vi "五参数水样测试.vi"(11 "启动参数":T1={"测量模式"=enum."水样测试", "数据标记表"="N", "测量时间"=3.0}) -> ()   [LabVIEW 2016, in "斯坦道仪器.lvlib"]
uses:
  PLC/PLC.lvlib
panel:
  out "枚举":T2(ring)
  out "状态":string
  out "数值":i32
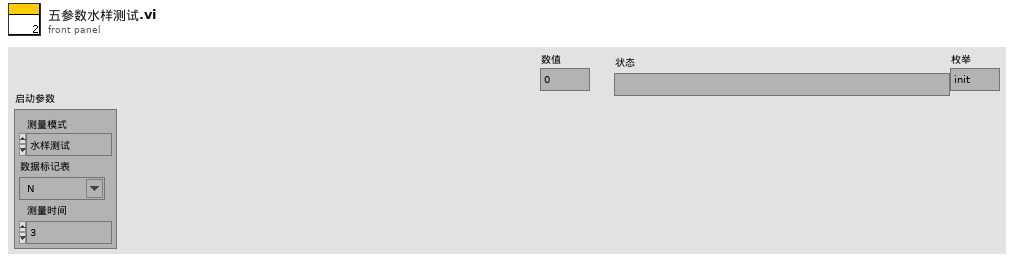
[diagram p1: front panel]
types:
  T1 = cluster{"测量模式":enum16{"待机", "水样测试", "标样核查", "零点核查", "跨度核查", "空白测试", "平行样测试", "加标回收", "空白校准", "标样校准", "初始化（清洗）"}, "数据标记表":string, "测量时间":dbl}
  T2 = enum16{"init", "开机", "启动测量", "读取测量值", "存储数据", "关闭测量", "关机", "结束"}
  T3 = cluster{"时间标识":timestamp, "设备":string, "日志信息":string, "流程参数":string}
  T4 = cluster{"starting address":u16, "holding register value":u16}
  T5 = enum16{"idle", "init", "读状态", "读参数", "多个写入", "单个写入", "线圈写入"}
  T6 = enum16{"待机", "水样测试", "标样核查", "零点核查", "跨度核查", "空白测试", "平行样测试", "加标回收", "空白校准", "标样校准", "初始化（清洗）"}
  T7 = cluster{"水温":dbl, "pH":dbl, "DO":dbl, "Cond":dbl, "Turb":dbl, "叶绿素":dbl, "藻密度":dbl, "蓝绿藻":dbl, "ORP":dbl, "NH3N":dbl}
  T8 = cluster{"数据标记表":string, "测量模式":enum16{"待机", "水样测试", "标样核查", "零点核查", "跨度核查", "空白测试", "平行样测试", "加标回收", "空白校准", "标样校准", "初始化（清洗）"}, "database":string}
  T9 = cluster{"因子编码":string, "单位":string, "标样参考值":sgl, "水样数据时间":timestamp, "水样实测值":sgl, "水样数据标识":string, "K":sgl, "B":sgl, "T":sgl, "H":sgl, "水深":sgl}
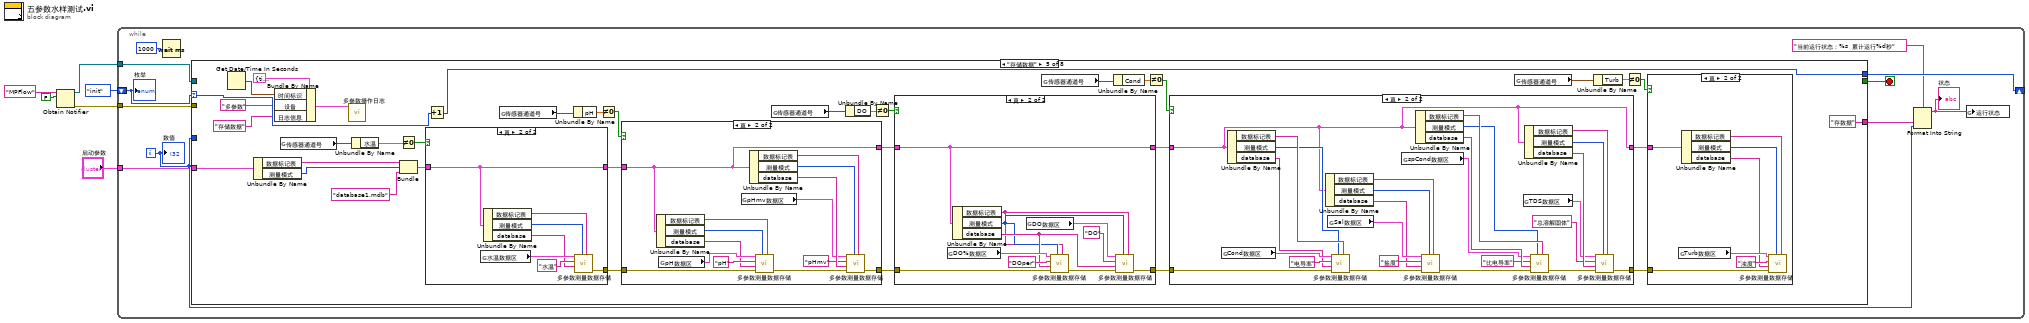
[diagram p0: block diagram]
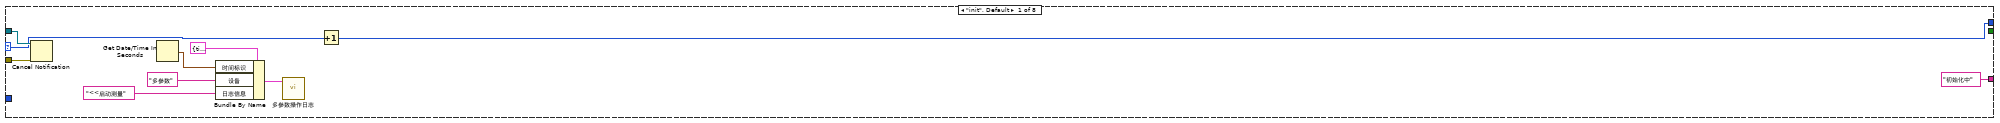
[diagram p2: hidden frame]
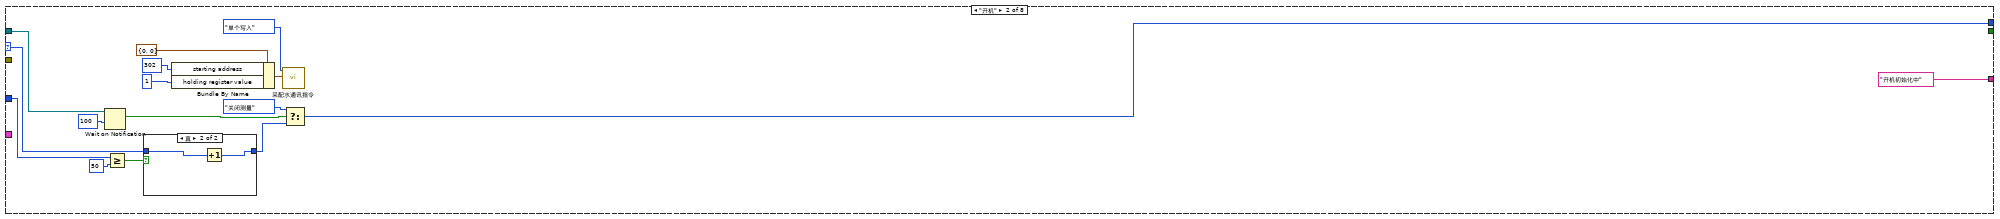
[diagram p3: hidden frame]
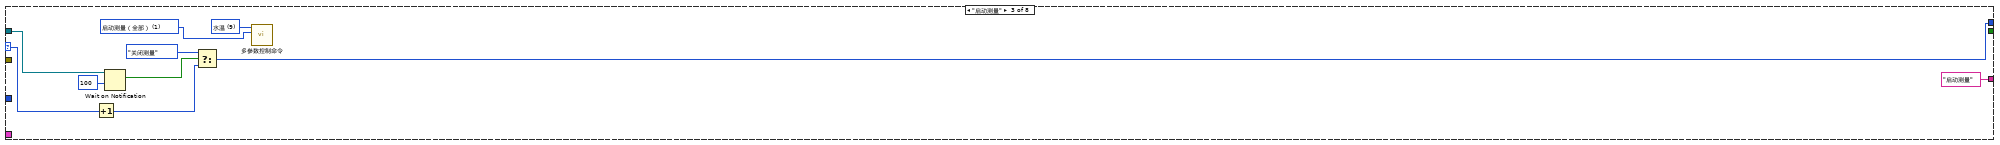
[diagram p5: hidden frame]
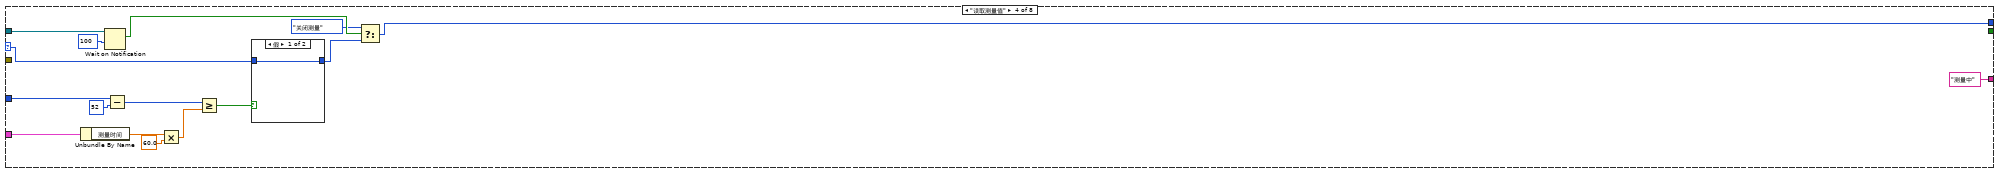
[diagram p6: hidden frame]
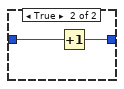
[diagram p7: hidden frame]
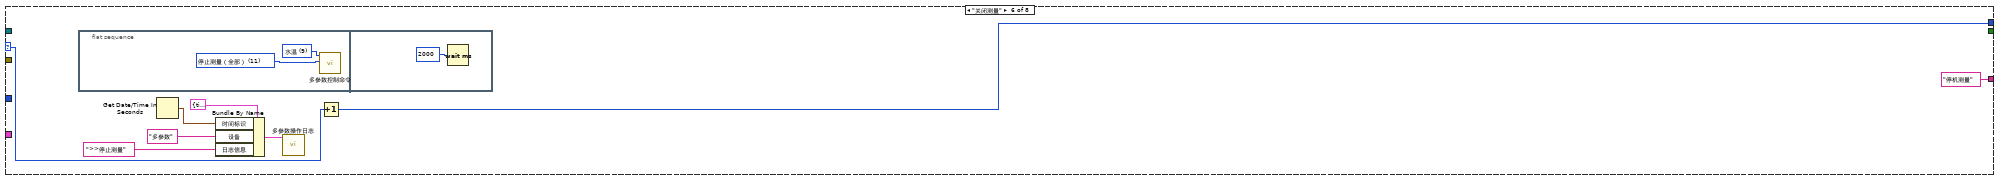
[diagram p13: hidden frame]
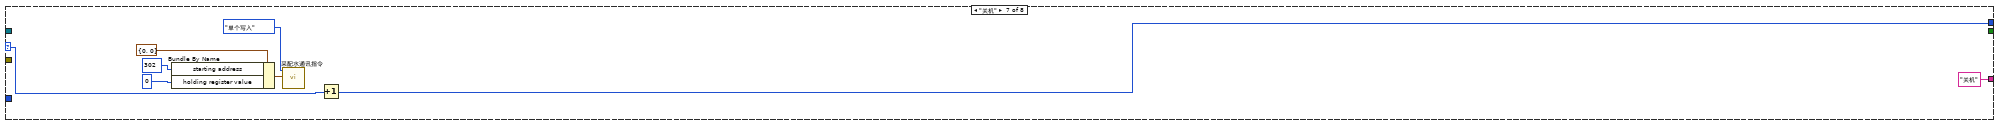
[diagram p14: hidden frame]
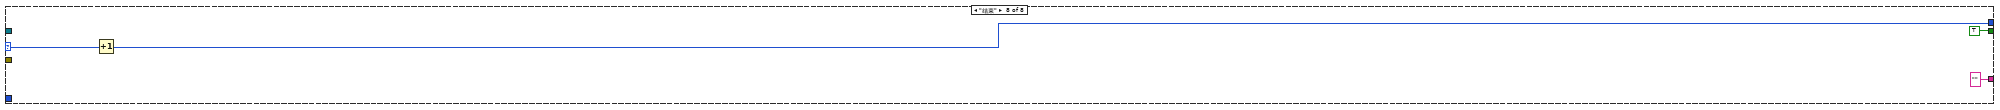
[diagram p15: hidden frame]
diagram:
  n1 = Obtain Notifier(name (unnamed)="MPFlow" ("名称（未命名）"), notification data type=FALSE) -> (notifier out=w3:refnum<notifier>, error out=w2:errorcluster)  [unwired: 2 in, 1 out]
  n2 = while {
    shift-right: [w13] -> _
    shift-left: T2."init" ("枚举") -> [w17]
    tunnel: w3 -> [w15]
    tunnel: w2 -> [w14]
    tunnel: "启动参数" -> [w7]
    i -> [w9]
    stop <- w16 stop-if-true
    n3 = Wait (ms)(milliseconds to wait=u32 1000 ("等待时间（毫秒）")) -> ()  [unwired: 1 out]
    n4 = case shown="\"存储数据\"" w17 {
      selector: w17 -> [w25 w38 w56 w72 w111 w188 w194 w202]
      tunnel: [_ _ _ _ _ _ _ TRUE] -> w16
      tunnel: w15 -> [w27 w33 w55 w69 _ _ _ _]
      tunnel: w14 -> [w26 _ _ _ _ _ _ _]
      tunnel: [w24 w31 w52 w67 w110 w187 w193 w201] -> w13
      tunnel: w9 -> [_ w37 _ w59 _ _ _ _]
      tunnel: ["初始化中" ("状态") "开机初始化中" ("状态") "启动测量" ("状态") "测量中" ("状态") "存数据" ("状态") "停机测量" ("状态") "关机" ("状态") "" ("状态")] -> w10
      tunnel: w7 -> [_ _ _ w63 w108 _ _ _]
      frame "init", Default {
        n5 = Cancel Notification(0:w27, 3:w26) -> ()  [unwired: 3 out]
        n6 = Get Date/Time In Seconds() -> (seconds since 1Jan1904=w21:timestamp)
        n7 = Bundle By Name(cluster=T3 {"时间标识"=timestamp(0 s since 1904-01-01), "设备"="", "日志信息"="", "流程参数"=""} ("data in"), "时间标识"=w21, "设备"="多参数", "日志信息"="<<启动测量") -> (w20:T3)
        n8 = call "多参数操作日志.vi"("data in"=w20) -> ()  [unwired: 10 in, 1 out]
        n9 = Increment(x=w25) -> (x+1=w24:T2)
      }
      frame "开机" {
        n10 = Wait on Notification(notifier=w33, timeout in ms (-1)=100 ("超时毫秒(-1)")) -> (notification=w34:bool)  [unwired: 2 in, 3 out]
        n11 = Greater Or Equal?(x=w37, y=50) -> (x >= y?=w35:bool)
        n12 = case shown="真" w35 {
          tunnel: w38 -> [w44 w46]
          tunnel: [w44 w45] -> w32
          frame False {
          }
          frame True {
            n13 = Increment(x=w46) -> (x+1=w45:T2)
          }
        }
        n14 = Bundle By Name(cluster=T4 {"starting address"=0, "holding register value"=0}, "starting address"=u16 302, "holding register value"=u16 1) -> (w41:T4)
        n15 = call "采配水通讯指令.vi"("数据"=w41, "命令"=T5."单个写入") -> ()  [unwired: 10 in]
        n16 = Select(t=T2."关闭测量" ("枚举"), s=w34, f=w32) -> (s? t:f=w31:T2)
      }
      frame "启动测量" {
        w47 = u16 1 items=["启动测量（全部）"=1, "初始化（清洗）"=10, "停止测量（全部）"=11, "校时"=13, "启动测量（单个传感器）"=19, "停止测量（单个传感器）"=20] ("控制命令")
        w48 = u16 9 items=["氨氮"=3, "水温"=9, "pH值"=10, "溶解氧"=11, "电导率"=12, "浊度"=13, "叶绿素a"=14, "藻密度"=15, "蓝绿藻"=16, "氧化还原电位"=17, "溶解氧%"=18, "盐度"=19] ("站号")
        n17 = Increment(x=w56) -> (x+1=w53:T2)
        n18 = Wait on Notification(notifier=w55, timeout in ms (-1)=100 ("超时毫秒(-1)")) -> (notification=w54:bool)  [unwired: 2 in, 3 out]
        n19 = Select(t=T2."关闭测量" ("枚举"), s=w54, f=w53) -> (s? t:f=w52:T2)
        n20 = call "多参数控制命令.vi"("控制命令"=w47, "站号"=w48) -> ()  [unwired: 9 in, 1 out]
      }
      frame "读取测量值" {
        n21 = Unbundle By Name(w63) -> ("测量时间"=w62:dbl)
        n22 = Wait on Notification(notifier=w69, timeout in ms (-1)=100 ("超时毫秒(-1)")) -> (notification=w70:bool)  [unwired: 2 in, 3 out]
        n23 = Subtract(x=w59, y=52) -> (x-y=w58:i32)
        n24 = Multiply(x=w62, y=60.0) -> (x*y=w60:dbl)
        n25 = Greater Or Equal?(x=w58, y=w60) -> (x >= y?=w71:bool)
        n26 = case shown="假" w71 {
          tunnel: w72 -> [w73 w75]
          tunnel: [w73 w74] -> w68
          frame False {
          }
          frame True {
            n27 = Increment(x=w75) -> (x+1=w74:T2)
          }
        }
        n28 = Select(t=T2."关闭测量" ("枚举"), s=w70, f=w68) -> (s? t:f=w67:T2)
      }
      frame "存储数据" {
        n29 = Get Date/Time In Seconds() -> (seconds since 1Jan1904=w79:timestamp)
        n30 = Unbundle By Name(w108) -> ("数据标记表"=w87:string, "测量模式"=w86:T6)
        n31 = Bundle By Name(cluster=T3 {"时间标识"=timestamp(0 s since 1904-01-01), "设备"="", "日志信息"="", "流程参数"=""} ("data in"), "时间标识"=w79, "设备"="多参数", "日志信息"="存储数据") -> (w78:T3)
        n32 = global read "多参数全局变量.vi" "传感器通道号"() -> (w103:T7)
        n33 = call "多参数操作日志.vi"("data in"=w78) -> ()  [unwired: 10 in, 1 out]
        n34 = Unbundle By Name(w103) -> ("水温"=w102:dbl)
        n35 = Not Equal To 0?(x=w102) -> (x != 0?=w101:bool)
        n36 = Bundle("数据标记表"=w87, "测量模式"=w86, "database"="database1.mdb") -> (w85:T8)  [unwired: 1 in]
        n37 = case shown="真" w101 {
          tunnel: [_ w178] -> w107
          tunnel: w85 -> [w173 w177]
          tunnel: [w173 w177] -> w84
          frame False {
          }
          frame True {
            n38 = global read "多参数全局变量.vi" "水温数据区"() -> (w180:T9)
            n39 = Unbundle By Name(w177) -> ("数据标记表"=w176:string, "测量模式"=w175:T6, "database"=w174:string)
            n40 = call "多参数测量数据存储.vi"("数据标记表"=w176, "测量模式"=w175, "database"=w174, "table输入"="水温", "data in"=w180) -> ("error out"=w178:errorcluster)  [unwired: 6 in]
          }
        }
        n41 = Increment(x=w111) -> (x+1=w110:T2)
        n42 = global read "多参数全局变量.vi" "传感器通道号"() -> (w96:T7)
        n43 = Unbundle By Name(w96) -> ("pH"=w95:dbl)
        n44 = Not Equal To 0?(x=w95) -> (x != 0?=w100:bool)
        n45 = case shown="真" w100 {
          tunnel: w107 -> [_ w172]
          tunnel: [_ w161] -> w106
          tunnel: w84 -> [w158 w166]
          tunnel: [w158 w166] -> w82
          frame False {
          }
          frame True {
            n46 = Unbundle By Name(w166) -> ("数据标记表"=w169:string, "测量模式"=w168:T6, "database"=w167:string)
            n47 = global read "多参数全局变量.vi" "pH数据区"() -> (w171:T9)
            n48 = global read "多参数全局变量.vi" "pHmv数据区"() -> (w160:T9)
            n49 = Unbundle By Name(w166) -> ("数据标记表"=w165:string, "测量模式"=w164:T6, "database"=w163:string)
            n50 = call "多参数测量数据存储.vi"("数据标记表"=w169, "测量模式"=w168, "error in (no error)"=w172, "database"=w167, "table输入"="pH", "data in"=w171) -> ("error out"=w162:errorcluster)  [unwired: 5 in]
            n51 = call "多参数测量数据存储.vi"("数据标记表"=w165, "测量模式"=w164, "error in (no error)"=w162, "database"=w163, "table输入"="pHmv", "data in"=w160) -> ("error out"=w161:errorcluster)  [unwired: 5 in]
          }
        }
        n52 = global read "多参数全局变量.vi" "传感器通道号"() -> (w94:T7)
        n53 = Unbundle By Name(w94) -> ("DO"=w93:dbl)
        n54 = Not Equal To 0?(x=w93) -> (x != 0?=w99:bool)
        n55 = case shown="真" w99 {
          tunnel: w106 -> [_ w157]
          tunnel: [_ w153] -> w105
          tunnel: [w146 w150] -> w83
          tunnel: w82 -> [w146 w150]
          frame False {
          }
          frame True {
            n56 = global read "多参数全局变量.vi" "DO%数据区"() -> (w152:T9)
            n57 = Unbundle By Name(w150) -> ("数据标记表"=w147:string, "测量模式"=w148:T6, "database"=w149:string)
            n58 = global read "多参数全局变量.vi" "DO数据区"() -> (w154:T9)
            n59 = call "多参数测量数据存储.vi"("数据标记表"=w147, "测量模式"=w148, "error in (no error)"=w157, "database"=w149, "table输入"="DOper", "data in"=w152) -> ("error out"=w156:errorcluster)  [unwired: 5 in]
            n60 = call "多参数测量数据存储.vi"("数据标记表"=w147, "测量模式"=w148, "error in (no error)"=w156, "database"=w149, "table输入"="DO", "data in"=w154) -> ("error out"=w153:errorcluster)  [unwired: 5 in]
          }
        }
        n61 = global read "多参数全局变量.vi" "传感器通道号"() -> (w92:T7)
        n62 = Unbundle By Name(w92) -> ("Cond"=w91:dbl)
        n63 = Not Equal To 0?(x=w91) -> (x != 0?=w98:bool)
        n64 = case shown="真" w98 {
          tunnel: w105 -> [_ w143]
          tunnel: [_ w124] -> w104
          tunnel: w83 -> [w119 w133]
          tunnel: [w119 w133] -> w81
          frame False {
          }
          frame True {
            n65 = global read "多参数全局变量.vi" "Cond数据区"() -> (w145:T9)
            n66 = Unbundle By Name(w133) -> ("数据标记表"=w138:string, "测量模式"=w137:T6, "database"=w139:string)
            n67 = Unbundle By Name(w133) -> ("数据标记表"=w136:string, "测量模式"=w135:T6, "database"=w134:string)
            n68 = global read "多参数全局变量.vi" "Sal数据区"() -> (w141:T9)
            n69 = call "多参数测量数据存储.vi"("数据标记表"=w138, "测量模式"=w137, "error in (no error)"=w143, "database"=w139, "table输入"="电导率", "data in"=w145) -> ("error out"=w142:errorcluster)  [unwired: 5 in]
            n70 = global read "多参数全局变量.vi" "spCond数据区"() -> (w123:T9)
            n71 = Unbundle By Name(w133) -> ("数据标记表"=w132:string, "测量模式"=w131:T6, "database"=w130:string)
            n72 = call "多参数测量数据存储.vi"("数据标记表"=w136, "测量模式"=w135, "error in (no error)"=w142, "database"=w134, "table输入"="盐度", "data in"=w141) -> ("error out"=w129:errorcluster)  [unwired: 5 in]
            n73 = global read "多参数全局变量.vi" "TDS数据区"() -> (w122:T9)
            n74 = Unbundle By Name(w133) -> ("数据标记表"=w125:string, "测量模式"=w126:T6, "database"=w127:string)
            n75 = call "多参数测量数据存储.vi"("数据标记表"=w132, "测量模式"=w131, "error in (no error)"=w129, "database"=w130, "table输入"="比电导率", "data in"=w123) -> ("error out"=w128:errorcluster)  [unwired: 5 in]
            n76 = call "多参数测量数据存储.vi"("数据标记表"=w125, "测量模式"=w126, "error in (no error)"=w128, "database"=w127, "table输入"="总溶解固体", "data in"=w122) -> ("error out"=w124:errorcluster)  [unwired: 5 in]
          }
        }
        n77 = global read "多参数全局变量.vi" "传感器通道号"() -> (w90:T7)
        n78 = Unbundle By Name(w90) -> ("Turb"=w89:dbl)
        n79 = Not Equal To 0?(x=w89) -> (x != 0?=w97:bool)
        n80 = case shown="真" w97 {
          tunnel: w104 -> [_ w118]
          tunnel: w81 -> [_ w115]
          frame False {
          }
          frame True {
            n81 = global read "多参数全局变量.vi" "Turb数据区"() -> (w117:T9)
            n82 = Unbundle By Name(w115) -> ("数据标记表"=w112:string, "测量模式"=w113:T6, "database"=w114:string)
            n83 = call "多参数测量数据存储.vi"("数据标记表"=w112, "测量模式"=w113, "error in (no error)"=w118, "database"=w114, "table输入"="浊度", "data in"=w117) -> ()  [unwired: 5 in, 1 out]
          }
        }
      }
      frame "关闭测量" {
        n84 = flat-sequence {
          frame #0 {
            w189 = u16 11 items=["启动测量（全部）"=1, "初始化（清洗）"=10, "停止测量（全部）"=11, "校时"=13, "启动测量（单个传感器）"=19, "停止测量（单个传感器）"=20] ("控制命令")
            w190 = u16 9 items=["氨氮"=3, "水温"=9, "pH值"=10, "溶解氧"=11, "电导率"=12, "浊度"=13, "叶绿素a"=14, "藻密度"=15, "蓝绿藻"=16, "氧化还原电位"=17, "溶解氧%"=18, "盐度"=19] ("站号")
            n85 = call "多参数控制命令.vi"("控制命令"=w189, "站号"=w190) -> ()  [unwired: 9 in, 1 out]
          }
          frame #1 {
            n86 = Wait (ms)(milliseconds to wait=u32 2000 ("等待时间（毫秒）")) -> ()  [unwired: 1 out]
          }
        }
        n87 = Get Date/Time In Seconds() -> (seconds since 1Jan1904=w184:timestamp)
        n88 = Bundle By Name(cluster=T3 {"时间标识"=timestamp(0 s since 1904-01-01), "设备"="", "日志信息"="", "流程参数"=""} ("data in"), "时间标识"=w184, "设备"="多参数", "日志信息"=">>停止测量") -> (w183:T3)
        n89 = call "多参数操作日志.vi"("data in"=w183) -> ()  [unwired: 10 in, 1 out]
        n90 = Increment(x=w188) -> (x+1=w187:T2)
      }
      frame "关机" {
        n91 = Bundle By Name(cluster=T4 {"starting address"=0, "holding register value"=0}, "starting address"=u16 302, "holding register value"=u16 0) -> (w197:T4)
        n92 = call "采配水通讯指令.vi"("数据"=w197, "命令"=T5."单个写入") -> ()  [unwired: 10 in]
        n93 = Increment(x=w194) -> (x+1=w193:T2)
      }
      frame "结束" {
        n94 = Increment(x=w202) -> (x+1=w201:T2)
      }
    }
    n95 = Format Into String(format string="当前运行状态：%s  累计运行%d秒" ("格式字符串"), w10, w9) -> (resulting string=w8:string)  [unwired: 2 in, 1 out]
    "状态" <- w8
    n96 = global write "多参数全局变量.vi" "运行状态"(w8) -> ()
    "数值" <- w9
    "枚举" <- w17
  }
